vi "Network Transceiver.vi"   [LabVIEW 2020]
uses:
  Type Definitions/Data Frame.ctl
  Type Definitions/Data Frame Header.ctl
  Type Definitions/Payload Class.ctl
  Type Definitions/Device.ctl
  Type Definitions/Device Parameters.ctl
  <vilib>/dex/Stream Element Allocation Mode.ctl
types:
  T1 = typedef "Device Parameters.ctl" = cluster{"Device":T2}
  T2 = typedef "Device.ctl" = enum32{"None", "Exec", "Aux1", "Aux2", "Aux3"}
  T3 = typedef "Data Frame.ctl" = cluster{"Frame Header":T4, "Payload":string, "CRC":u32}
  T4 = typedef "Data Frame Header.ctl" = cluster{"Sync":u32, "Time":dbl, "Nanosecond Counter":i64, "Payload Class":T5, "Payload ID":u16, "Counter":i32, "Options":u32, "Source":T2, "Destination":T2}
  T5 = typedef "Payload Class.ctl" = enum16{"System State", "Parameters", "Metadata", "Software Monitor", "Data", "Commands"}
  T6 = typedef "Stream Element Allocation Mode.ctl" = u32
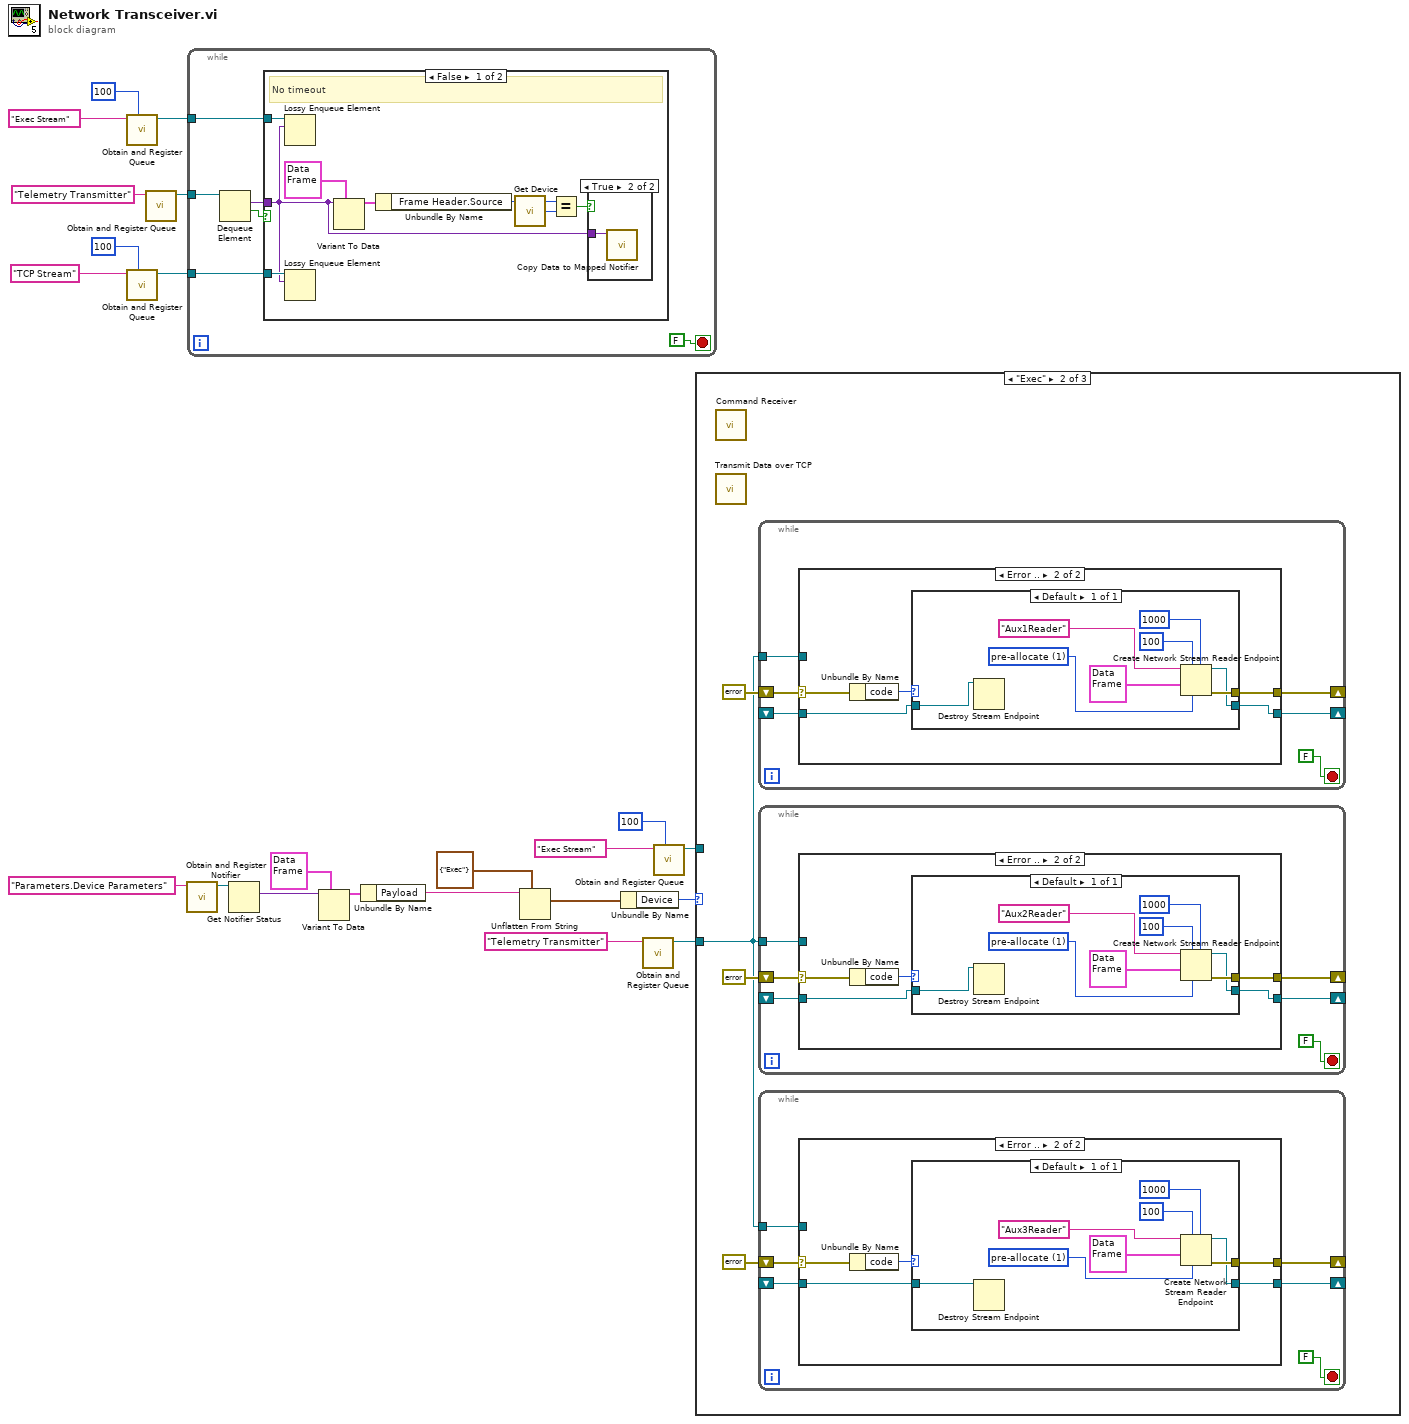
[diagram p0: block diagram]
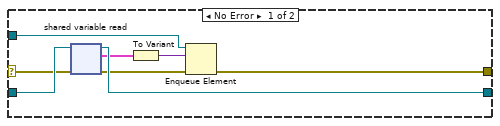
[diagram p5: hidden frame]
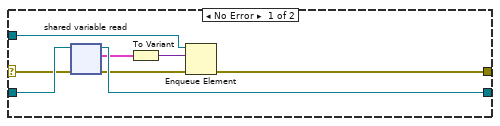
[diagram p6: hidden frame]
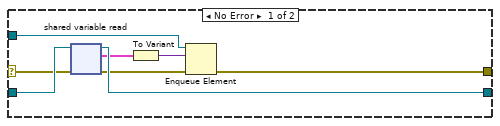
[diagram p7: hidden frame]
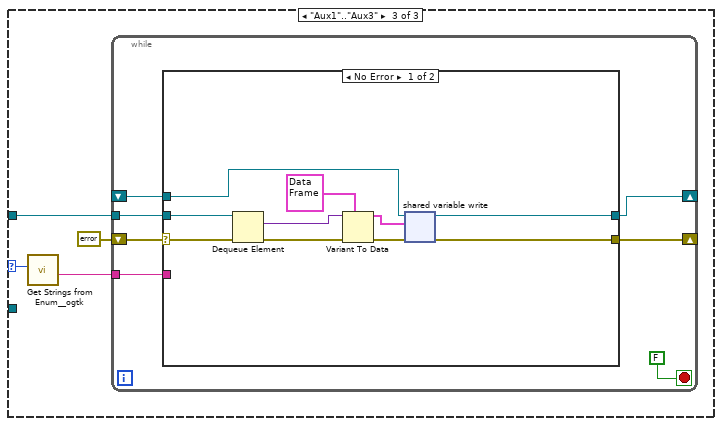
[diagram p8: hidden frame]
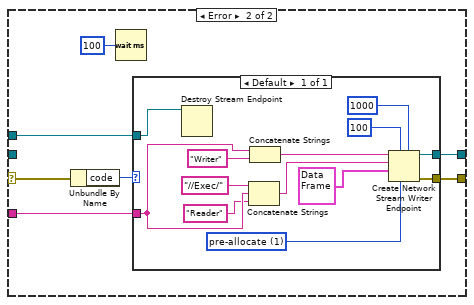
[diagram p9: hidden frame]
diagram:
  n1 = call "Obtain and Register Queue.vi"("max queue size (-1, unlimited)"=100, "name (unnamed)"="Exec Stream") -> ("Queue Out"=w6:refnum<queue>)  [unwired: 6 in, 3 out]
  n2 = call "Obtain and Register Queue.vi"("max queue size (-1, unlimited)"=100, "name (unnamed)"="TCP Stream") -> ("Queue Out"=w12:refnum<queue>)  [unwired: 6 in, 3 out]
  n3 = call "Obtain and Register Queue.vi"("name (unnamed)"="Telemetry Transmitter") -> ("Queue Out"=w13:refnum<queue>)  [unwired: 7 in, 3 out]
  n4 = call "Obtain and Register Notifier.vi"("name (unnamed)"="Parameters.Device Parameters") -> ("notifier out"=w21:refnum<notifier>)  [unwired: 8 in, 2 out]
  n5 = while {
    tunnel: w13 -> [w28]
    tunnel: w12 -> [w26]
    tunnel: w6 -> [w23]
    stop <- FALSE stop-if-true
    n6 = Dequeue Element(queue=w28) -> (element=w25:variant, timed out?=w24:bool)  [unwired: 2 in, 2 out]
    n7 = case shown="False" w24 {
      tunnel: w26 -> [w36 _]
      tunnel: w25 -> [w29 _]
      tunnel: w23 -> [w35 _]
      frame False {
        # "No timeout"
        n8 = Lossy Enqueue Element(queue=w35, element=w29) -> ()  [unwired: 1 in, 4 out]
        n9 = Lossy Enqueue Element(queue=w36, element=w29) -> ()  [unwired: 1 in, 4 out]
        n10 = Variant To Data(type=T3 {"Frame Header"={"Sync"=0, "Time"=0.0, "Nanosecond Counter"=0, "Payload Class"=enum."System State", "Payload ID"=0, "Counter"=0, "Options"=0, "Source"=enum."None", "Destination"=enum."None"}, "Payload"="", "CRC"=0} ("Frame"), Variant=w29) -> (data=w33:T3)  [unwired: 1 in, 1 out]
        n11 = Unbundle By Name(w33) -> ("Frame Header.Source"=w32:T2)
        n12 = call "Get Device.vi"() -> ("Device"=w31:T2)  [unwired: 5 in]
        n13 = Equal?(x=w32, y=w31) -> (x = y?=w30:bool)
        n14 = case shown="True" w30 {
          tunnel: w29 -> [_ w37]
          frame False {
          }
          frame True {
            n15 = call "Copy Data to Mapped Notifier.vi"("Variant"=w37) -> ()  [unwired: 11 in]
          }
        }
      }
      frame True {
        # "Timed out"
      }
    }
  }
  n16 = Get Notifier Status(notifier=w21) -> (current notification=w20:variant)  [unwired: 1 in, 4 out]
  n17 = Variant To Data(type=T3 {"Frame Header"={"Sync"=0, "Time"=0.0, "Nanosecond Counter"=0, "Payload Class"=enum."System State", "Payload ID"=0, "Counter"=0, "Options"=0, "Source"=enum."None", "Destination"=enum."None"}, "Payload"="", "CRC"=0} ("Frame"), Variant=w20) -> (data=w18:T3)  [unwired: 1 in, 1 out]
  n18 = Unbundle By Name(w18) -> ("Payload"=w17:string)
  n19 = Unflatten From String(type=T1 {"Device"=enum."Exec"} ("Device Parameters"), binary string=w17) -> (value=w15:T1)  [unwired: 3 in, 2 out]
  n20 = Unbundle By Name(w15) -> ("Device"=w14:T2)
  n21 = call "Obtain and Register Queue.vi"("name (unnamed)"="Telemetry Transmitter") -> ("Queue Out"=w1:refnum<queue>)  [unwired: 7 in, 3 out]
  n22 = call "Obtain and Register Queue.vi"("max queue size (-1, unlimited)"=100, "name (unnamed)"="Exec Stream") -> ("Queue Out"=w3:refnum<queue>)  [unwired: 6 in, 3 out]
  n23 = case shown="\"Exec\"" w14 {
    selector: w14 -> [_ _ w125]
    tunnel: w3 -> [_ _ w123]
    tunnel: w1 -> [_ w38 _]
    frame "None", Default {
    }
    frame "Exec" {
      n24 = call "Command Receiver.vi"() -> ()  [unwired: 12 in]
      n25 = call "Transmit Data over TCP.vi"() -> ()  [unwired: 12 in]
      n26 = while {
        shift-right: [w101] -> _
        shift-left: errorcluster {"status"=TRUE, "code"=0, "source"=""} ("error out") -> [w100]
        shift-right: [w99] -> _
        shift-left: _ -> [w98]
        tunnel: w38 -> [w96]
        stop <- FALSE stop-if-true
        n27 = case shown="Error .." w100 {
          selector: w100 -> [w107 w112]
          tunnel: [w105 w114] -> w101
          tunnel: [w108 w113] -> w99
          tunnel: w98 -> [w109 w110]
          tunnel: w96 -> [w104 _]
          frame No Error {
            n28 = shared-variable-read(w109, w107) -> (w108:refnum<k21>, w106:errorcluster, w103:T3)  [unwired: 1 in, 1 out]
            n29 = To Variant(anything=w103) -> (Variant=w102:variant)
            n30 = Enqueue Element(queue=w104, element=w102, error in (no error)=w106) -> (error out=w105:errorcluster)  [unwired: 1 in, 2 out]
          }
          frame Error {
            n31 = Unbundle By Name(w112) -> ("code"=w111:i32)
            n32 = case shown="Default" w111 {
              tunnel: [w122] -> w114
              tunnel: [w116] -> w113
              tunnel: w110 -> [w115]
              frame Default {
                w118 = T6 1 items=["allocate as needed", "pre-allocate"] ("element allocation mode")
                n33 = Destroy Stream Endpoint(11:w115) -> ()  [unwired: 1 in, 1 out]
                n34 = Create Network Stream Reader Endpoint(5:1000 ("timeout in ms (-1)"), 6:w118, 7:100 ("reader buffer size"), 9:T3 {"Frame Header"={"Sync"=0, "Time"=0.0, "Nanosecond Counter"=0, "Payload Class"=enum."System State", "Payload ID"=0, "Counter"=0, "Options"=0, "Source"=enum."None", "Destination"=enum."None"}, "Payload"="", "CRC"=0} ("Frame"), 11:"Aux1Reader" ("reader name")) -> (0:w122:errorcluster, 3:w116:refnum<k21>)  [unwired: 2 in]
              }
            }
          }
        }
      }
      n35 = while {
        shift-right: [w74] -> _
        shift-left: errorcluster {"status"=TRUE, "code"=0, "source"=""} ("error out") -> [w73]
        shift-right: [w72] -> _
        shift-left: _ -> [w71]
        tunnel: w38 -> [w69]
        stop <- FALSE stop-if-true
        n36 = case shown="Error .." w73 {
          selector: w73 -> [w80 w85]
          tunnel: [w78 w87] -> w74
          tunnel: [w81 w86] -> w72
          tunnel: w71 -> [w82 w83]
          tunnel: w69 -> [w77 _]
          frame No Error {
            n37 = shared-variable-read(w82, w80) -> (w81:refnum<k21>, w79:errorcluster, w76:T3)  [unwired: 1 in, 1 out]
            n38 = To Variant(anything=w76) -> (Variant=w75:variant)
            n39 = Enqueue Element(queue=w77, element=w75, error in (no error)=w79) -> (error out=w78:errorcluster)  [unwired: 1 in, 2 out]
          }
          frame Error {
            n40 = Unbundle By Name(w85) -> ("code"=w84:i32)
            n41 = case shown="Default" w84 {
              tunnel: [w95] -> w87
              tunnel: [w89] -> w86
              tunnel: w83 -> [w88]
              frame Default {
                w91 = T6 1 items=["allocate as needed", "pre-allocate"] ("element allocation mode")
                n42 = Destroy Stream Endpoint(11:w88) -> ()  [unwired: 1 in, 1 out]
                n43 = Create Network Stream Reader Endpoint(5:1000 ("timeout in ms (-1)"), 6:w91, 7:100 ("reader buffer size"), 9:T3 {"Frame Header"={"Sync"=0, "Time"=0.0, "Nanosecond Counter"=0, "Payload Class"=enum."System State", "Payload ID"=0, "Counter"=0, "Options"=0, "Source"=enum."None", "Destination"=enum."None"}, "Payload"="", "CRC"=0} ("Frame"), 11:"Aux2Reader" ("reader name")) -> (0:w95:errorcluster, 3:w89:refnum<k21>)  [unwired: 2 in]
              }
            }
          }
        }
      }
      n44 = while {
        shift-right: [w47] -> _
        shift-left: errorcluster {"status"=TRUE, "code"=0, "source"=""} ("error out") -> [w46]
        shift-right: [w45] -> _
        shift-left: _ -> [w44]
        tunnel: w38 -> [w42]
        stop <- FALSE stop-if-true
        n45 = case shown="Error .." w46 {
          selector: w46 -> [w53 w58]
          tunnel: [w51 w60] -> w47
          tunnel: [w54 w59] -> w45
          tunnel: w44 -> [w55 w56]
          tunnel: w42 -> [w50 _]
          frame No Error {
            n46 = shared-variable-read(w55, w53) -> (w54:refnum<k21>, w52:errorcluster, w49:T3)  [unwired: 1 in, 1 out]
            n47 = To Variant(anything=w49) -> (Variant=w48:variant)
            n48 = Enqueue Element(queue=w50, element=w48, error in (no error)=w52) -> (error out=w51:errorcluster)  [unwired: 1 in, 2 out]
          }
          frame Error {
            n49 = Unbundle By Name(w58) -> ("code"=w57:i32)
            n50 = case shown="Default" w57 {
              tunnel: [w68] -> w60
              tunnel: [w62] -> w59
              tunnel: w56 -> [w61]
              frame Default {
                w64 = T6 1 items=["allocate as needed", "pre-allocate"] ("element allocation mode")
                n51 = Destroy Stream Endpoint(11:w61) -> ()  [unwired: 1 in, 1 out]
                n52 = Create Network Stream Reader Endpoint(5:1000 ("timeout in ms (-1)"), 6:w64, 7:100 ("reader buffer size"), 9:T3 {"Frame Header"={"Sync"=0, "Time"=0.0, "Nanosecond Counter"=0, "Payload Class"=enum."System State", "Payload ID"=0, "Counter"=0, "Options"=0, "Source"=enum."None", "Destination"=enum."None"}, "Payload"="", "CRC"=0} ("Frame"), 11:"Aux3Reader" ("reader name")) -> (0:w68:errorcluster, 3:w62:refnum<k21>)  [unwired: 2 in]
              }
            }
          }
        }
      }
    }
    frame "Aux1".."Aux3" {
      n53 = call <userlib>:"Get Strings from Enum__ogtk.vi"("Enum"=w125) -> ("String Value"=w124:string)  [unwired: 7 in, 3 out]
      n54 = while {
        shift-right: [w133] -> _
        shift-left: errorcluster {"status"=TRUE, "code"=0, "source"=""} ("error out") -> [w132]
        shift-right: [w131] -> _
        shift-left: _ -> [w130]
        tunnel: w124 -> [w128]
        tunnel: w123 -> [w127]
        stop <- FALSE stop-if-true
        n55 = case shown="No Error" w132 {
          selector: w132 -> [w134 w148]
          tunnel: [w141 w150] -> w133
          tunnel: [w142 w149] -> w131
          tunnel: w130 -> [w143 w146]
          tunnel: w128 -> [_ w145]
          tunnel: w127 -> [w140 _]
          frame No Error {
            n56 = Dequeue Element(queue=w140, error in (no error)=w134) -> (element=w139:variant, error out=w135:errorcluster)  [unwired: 1 in, 2 out]
            n57 = Variant To Data(error in=w135, type=T3 {"Frame Header"={"Sync"=0, "Time"=0.0, "Nanosecond Counter"=0, "Payload Class"=enum."System State", "Payload ID"=0, "Counter"=0, "Options"=0, "Source"=enum."None", "Destination"=enum."None"}, "Payload"="", "CRC"=0} ("Frame"), Variant=w139) -> (data=w137:T3, error out=w136:errorcluster)
            n58 = shared-variable-write(w143, w136, w137) -> (w142:refnum<k21>, w141:errorcluster)  [unwired: 1 in, 1 out]
          }
          frame Error {
            n59 = Unbundle By Name(w148) -> ("code"=w147:i32)
            n60 = Wait (ms)(milliseconds to wait=u32 100) -> ()  [unwired: 1 out]
            n61 = case shown="Default" w147 {
              tunnel: [w158] -> w150
              tunnel: [w159] -> w149
              tunnel: w146 -> [w157]
              tunnel: w145 -> [w153]
              frame Default {
                w162 = T6 1 items=["allocate as needed", "pre-allocate"] ("element allocation mode")
                n62 = Destroy Stream Endpoint(11:w157) -> ()  [unwired: 1 in, 1 out]
                n63 = Concatenate Strings("//Exec/" ("string"), w153, "Reader" ("string")) -> (w151:string)
                n64 = Concatenate Strings(w153, "Writer" ("string")) -> (w155:string)
                n65 = Create Network Stream Writer Endpoint(5:1000 ("timeout in ms (-1)"), 6:w162, 7:100 ("reader buffer size"), 9:T3 {"Frame Header"={"Sync"=0, "Time"=0.0, "Nanosecond Counter"=0, "Payload Class"=enum."System State", "Payload ID"=0, "Counter"=0, "Options"=0, "Source"=enum."None", "Destination"=enum."None"}, "Payload"="", "CRC"=0} ("Frame"), 10:w151, 11:w155) -> (0:w158:errorcluster, 3:w159:refnum<k21>)  [unwired: 1 in]
              }
            }
          }
        }
      }
    }
  }
